vi "Start Trigger.vi"(8 "error in (no error)":errorcluster, 10 "Params":variant, 11 "NI DMM in":refnum<class "NI DMM.lvclass">) -> (0 "error out":errorcluster, 3 "NI DMM out":refnum<class "NI DMM.lvclass">)   [LabVIEW 2020, in "NI DMM.lvlib" / "NI DMM.lvclass"]
uses:
  NI DMM.lvclass
  TypeDefs/Trigger settings.ctl
  <instrlib>/niDMM/nidmm.llb/niDMM Trigger.ctl
  <instrlib>/niDMM/nidmm.llb/niDMM Slope.ctl
  NI DMM.lvclass/NI DMM.ctl
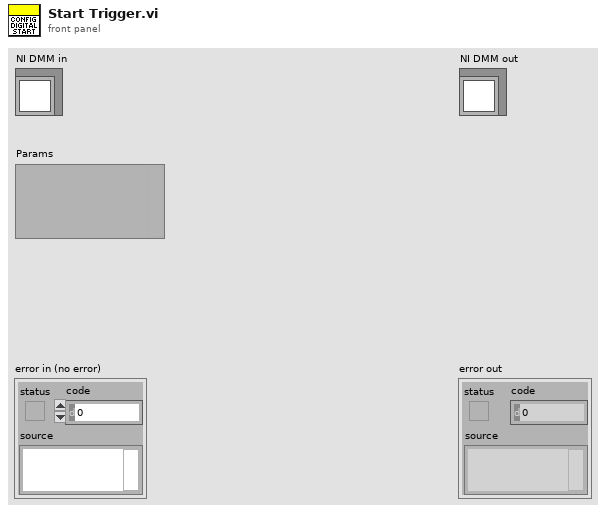
[diagram p1: front panel]
types:
  T1 = typedef "Trigger settings.ctl" = cluster{"Trigger Source":T2, "Trigger Delay (sec)":dbl, "Slope":T3}
  T2 = typedef "niDMM Trigger.ctl" = enum16{"Immediate", "External", "TTL 0", "TTL 1", "TTL 2", "TTL 3", "TTL 4", "TTL 5", "TTL 6", "Software", "TTL 7", "PXI Star", "LBR Trig 1", "Aux Trig 1"}
  T3 = typedef "niDMM Slope.ctl" = enum16{"Rising Edge", "Falling Edge"}
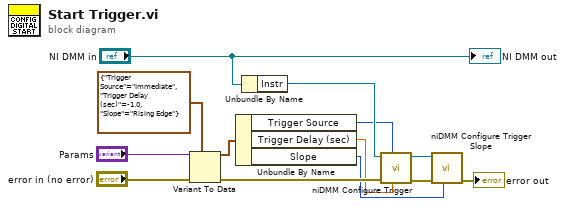
[diagram p0: block diagram]
diagram:
  n1 = Variant To Data(error in="error in (no error)", type=T1 {"Trigger Source"=enum."Immediate", "Trigger Delay (sec)"=-1.0, "Slope"=enum."Rising Edge"}, Variant="Params") -> (data=w6:T1, error out=w10:errorcluster)
  n2 = Unbundle By Name(w6) -> ("Trigger Source"=w3:T2, "Trigger Delay (sec)"=w2:dbl, "Slope"=w1:T3)
  n3 = Unbundle By Name("NI DMM in") -> ("Instr"=w4:refnum<k15>)
  n4 = call <instrlib>:"niDMM Configure Trigger.vi"("Trigger Delay (sec)"=w2, "Trigger Source"=w3, "error in (no error)"=w10, "instrument handle"=w4) -> ("error out"=w13:errorcluster, "instrument handle out"=w12:refnum<k15>)  [unwired: 6 in]
  n5 = call <instrlib>:"niDMM Configure Trigger Slope.vi"("Slope"=w1, "error in (no error)"=w13, "instrument handle"=w12) -> ("error out"=→"error out":errorcluster)  [unwired: 7 in, 1 out]
  "NI DMM out" <- "NI DMM in"
